vi "Scope.vi"(8 "error in (no error)":errorcluster, 11 "DAQmx in":refnum<class "DAQmx.lvclass">) -> (0 "error out":errorcluster, 3 "DAQmx out":refnum<class "DAQmx.lvclass">)   [LabVIEW 2019, in "DAQmx.lvclass"]
uses:
  DAQmx.lvclass
  DAQmx.lvclass/DAQmx.ctl
panel:
  in  "AO and AI index":i32
  out "t0":timestamp[](array[timestamp]) format="%<%.2X>T"
  out "Waveform Graph":waveform(dbl)[](graph)
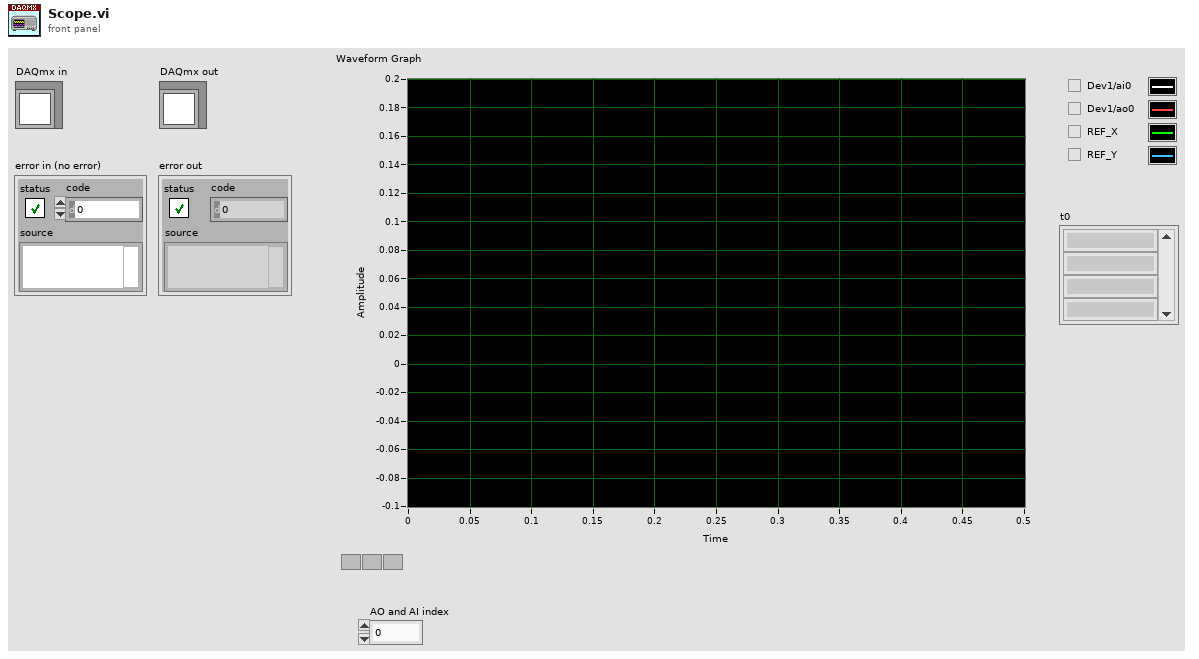
[diagram p1: front panel]
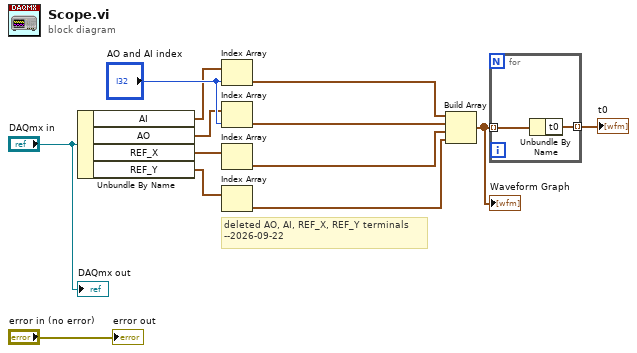
[diagram p0: block diagram]
diagram:
  # "deleted AO, AI, REF_X, REF_Y terminals\n--2026-09-22"
  n1 = Unbundle By Name("DAQmx in") -> ("AI"=w6:waveform(dbl)[], "AO"=w5:waveform(dbl)[], "REF_X"=w4:waveform(dbl)[], "REF_Y"=w3:waveform(dbl)[])
  n2 = Index Array(array=w6, index="AO and AI index") -> (element=w10:waveform(dbl))
  n3 = Index Array(array=w5, index="AO and AI index") -> (element=w9:waveform(dbl))
  n4 = Index Array(array=w4) -> (element=w13:waveform(dbl))  [unwired: 1 in]
  n5 = Index Array(array=w3) -> (element=w12:waveform(dbl))  [unwired: 1 in]
  n6 = Build Array(w10, w9, w13, w12) -> (w7:waveform(dbl)[])
  "Waveform Graph" <- w7
  n7 = for {
    tunnel: w7 -> [w15] mode=indexing
    tunnel: [w14] -> w11 mode=indexing
    n8 = Unbundle By Name(w15) -> ("t0"=w14:timestamp)
  }
  "t0" <- w11
  "error out" <- "error in (no error)"
  "DAQmx out" <- "DAQmx in"
